vi "GameConfig_update.vi"() -> ()   [LabVIEW 2017]
uses:
  GameConfig_data.ctl
  <vilib>/Utility/config.llb/NI_LVConfig.lvlib
panel:
  in  "cancel":bool
  in  "ok":bool
  in  "GameConfig":T1={"SpaceShip"={"Angle"=15.0, "SideLenght"=40.0, "MaxLinearVeloc"=250.0, "MaxAngularVeloc"=100.0, "LinearAceleration"=200.0, "AngularAceleration"=200.0}, "Physics"={"LinearDragFactor"=0.9, "AngularDragFactor"=0.9}, "Asteroids"={"MaxSize"=100.0, "MaxDivisions"=3, "MaxVeloc"=200.0, "MinVeloc"=50.0, "Fill"=TRUE}, "Environment"={"MaxAsteroids"=10, "TimeIncrement"=0.1, "AsterProbCreation"=0.5, "LogEnabled"=TRUE}, "Shots"={"MinTimeShots"=0.1, "ShotSize"=5.0, "ShotSpeed"=500.0}} {"Shots"."MinTimeShots" format="%.2f"}
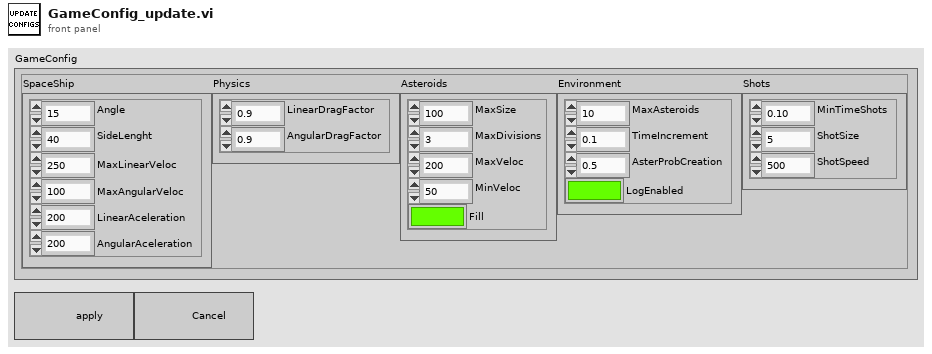
[diagram p1: front panel]
types:
  T1 = typedef "GameConfig_data.ctl" = cluster{"SpaceShip":cluster{"Angle":dbl, "SideLenght":dbl, "MaxLinearVeloc":dbl, "MaxAngularVeloc":dbl, "LinearAceleration":dbl, "AngularAceleration":dbl}, "Physics":cluster{"LinearDragFactor":dbl, "AngularDragFactor":dbl}, "Asteroids":cluster{"MaxSize":dbl, "MaxDivisions":i32, "MaxVeloc":dbl, "MinVeloc":dbl, "Fill":bool}, "Environment":cluster{"MaxAsteroids":i32, "TimeIncrement":dbl, "AsterProbCreation":dbl, "LogEnabled":bool}, "Shots":cluster{"MinTimeShots":dbl, "ShotSize":dbl, "ShotSpeed":dbl}}
  T2 = typedef "NI_LVConfig.lvlib/Config Data RefNum.ctl" = refnum<k1>
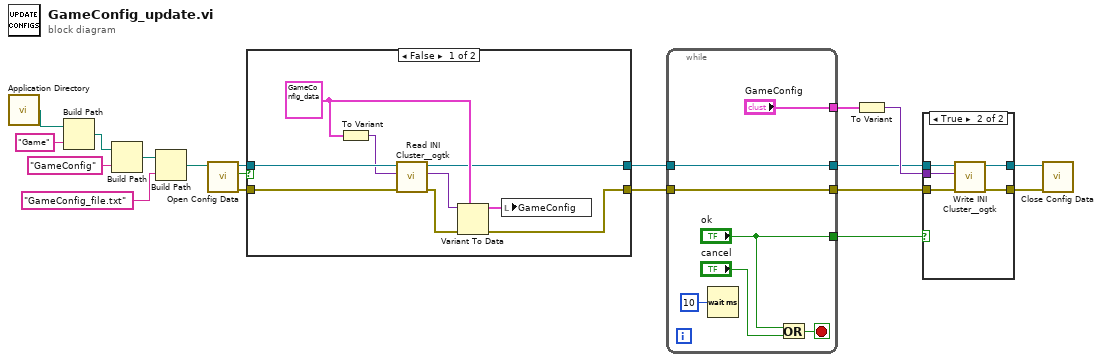
[diagram p0: block diagram]
diagram:
  n1 = call <vilib>:"Application Directory.vi"() -> ("Application Directory"=w10:path)
  n2 = Build Path(base path=w10, name or relative path="Game") -> (appended path=w11:path)
  n3 = Build Path(base path=w11, name or relative path="GameConfig") -> (appended path=w18:path)
  n4 = Build Path(base path=w18, name or relative path="GameConfig_file.txt") -> (appended path=w16:path)
  n5 = call <vilib>:"Open Config Data.vi"("configuration file path"=w16) -> ("error out"=w8:errorcluster, "file created?"=w9:bool, "refnum"=w7:T2)  [unwired: 8 in]
  n6 = case shown="False" w9 {
    tunnel: w8 -> [w28 w29]
    tunnel: w7 -> [w27 w30]
    tunnel: [w21 w29] -> w5
    tunnel: [w20 w30] -> w2
    frame False {
      w23 = T1 {"SpaceShip"={"Angle"=30.0, "SideLenght"=2.0, "MaxLinearVeloc"=10.0, "MaxAngularVeloc"=10.0, "LinearAceleration"=1.0, "AngularAceleration"=1.0}, "Physics"={"LinearDragFactor"=1.0, "AngularDragFactor"=1.0}, "Asteroids"={"MaxSize"=6.0, "MaxDivisions"=3, "MaxVeloc"=8.0, "MinVeloc"=1.0, "Fill"=FALSE}, "Environment"={"MaxAsteroids"=10, "TimeIncrement"=0.1, "AsterProbCreation"=0.1, "LogEnabled"=FALSE}, "Shots"={"MinTimeShots"=10.0, "ShotSize"=0.1, "ShotSpeed"=0.1}} ("GameConfig_data")
      n7 = To Variant(anything=w23) -> (Variant=w26:variant)
      n8 = call <userlib>:"Read INI Cluster__ogtk.vi"("error in (no error)"=w28, "INI Fomatted Cluster Type"=w26, "refnum"=w27) -> ("error out"=w25:errorcluster, "INI Fomatted Cluster"=w24:variant, "dup refnum"=w20:T2)  [unwired: 4 in, 2 out]
      n9 = Variant To Data(error in=w25, type=w23, Variant=w24) -> (data=w22:T1, error out=w21:errorcluster)
      n10 = local write "GameConfig"(w22) -> ()
    }
    frame True {
    }
  }
  n11 = while {
    tunnel: ["GameConfig"] -> w6
    tunnel: w5 -> [w33]
    tunnel: [w33] -> w4
    tunnel: [w32] -> w3
    tunnel: w2 -> [w32]
    tunnel: ["ok"] -> w1
    stop <- w34 stop-if-true
    n12 = Wait (ms)(milliseconds to wait=u32 10) -> ()  [unwired: 1 out]
    n13 = Or(x="ok", y="cancel") -> (x .or. y?=w34:bool)
  }
  n14 = To Variant(anything=w6) -> (Variant=w15:variant)
  n15 = case shown="True" w1 {
    tunnel: w15 -> [_ w44]
    tunnel: [w38 w43] -> w14
    tunnel: [w39 w42] -> w13
    tunnel: w4 -> [w38 w41]
    tunnel: w3 -> [w39 w40]
    frame False {
    }
    frame True {
      n16 = call <userlib>:"Write INI Cluster__ogtk.vi"("error in (no error)"=w41, "INI Fomatted Cluster"=w44, "refnum"=w40) -> ("error out"=w43:errorcluster, "dup refnum"=w42:T2)  [unwired: 7 in]
    }
  }
  n17 = call <vilib>:"Close Config Data.vi"("error in (no error)"=w14, "refnum"=w13) -> ()  [unwired: 8 in, 2 out]
